vi "Add Row to Database.vi"(8 "error in (no error)":errorcluster, 10 "Form ID":T1, 11 "Form Server in":refnum<class "Form Server.lvclass">) -> (0 "error out":errorcluster, 3 "Form Server out":refnum<class "Form Server.lvclass">)   [LabVIEW 2020, in "Form Server.lvlib" / "Form Server.lvclass"]
uses:
  Form Server.lvclass
  Autoclose manager/Form ID.ctl
  Form Server.lvclass/Form Server.ctl
  <vilib>/ActorFramework/Message Enqueuer/Message Enqueuer.lvclass/Message Enqueuer.ctl
  <vilib>/ActorFramework/Message Enqueuer/Enqueue.vi
  Forms Model/Form Model Interfaces/Form Model Messages Messages/Add row to database Msg/Add row to database Msg.lvclass
  C:/Program Files (x86)/National Instruments/LabVIEW 2020/vi.lib/ActorFramework/Message/Message.lvclass
  <vilib>/ActorFramework/Message Priority Queue/Priority Enqueue.vi
  Form Server Interfaces.lvlib
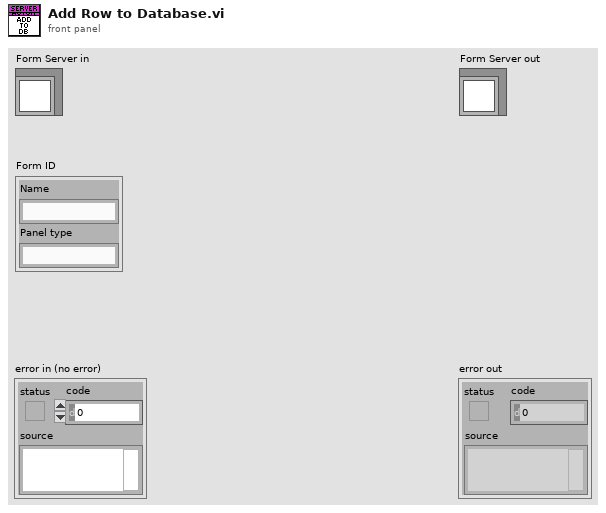
[diagram p1: front panel]
types:
  T1 = typedef "Form Server Interfaces.lvlib/Form ID.ctl" = cluster{"Name":string, "Panel type":string}
  T2 = map{T1, refnum<class "Message Enqueuer.lvclass">}
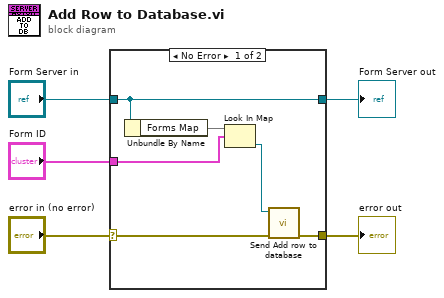
[diagram p0: block diagram]
diagram:
  n1 = case shown="No Error" "error in (no error)" {
    selector: "error in (no error)" -> [w11 w13]
    tunnel: [w10 w13] -> w4
    tunnel: "Form Server in" -> [w6 w12]
    tunnel: [w6 w12] -> w2
    tunnel: "Form ID" -> [w8 _]
    frame No Error {
      n2 = Unbundle By Name(w6) -> ("Forms Map"=w9:T2)
      n3 = Look In Map(map=w9, key=w8) -> (value=w7:refnum<class "Message Enqueuer.lvclass">)  [unwired: 1 in, 1 out]
      n4 = call "Send Add row to database.vi"("error in (no error)"=w11, "Message Enqueuer"=w7) -> ("error out"=w10:errorcluster)  [unwired: 8 in, 1 out]
    }
    frame Error {
    }
  }
  "error out" <- w4
  "Form Server out" <- w2
